vi "tsdiag_can_read_data_by_identifier.vi"(8 "error in (no error)":errorcluster, 9 "ADataIdentifier":u16 format="%.0x", 10 "ADiagModuleIndex":i32, 11 "路径输入":path) -> (0 "error out":errorcluster, 1 "Data":u8[](array[numeric]), 2 "return":i32, 3 "路径输出":path)   [LabVIEW 2014]
doc: "22服务，根据ID读取数据。"
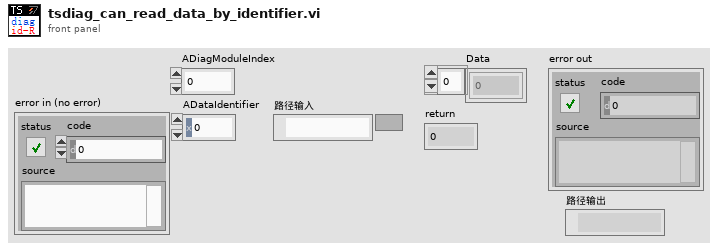
[diagram p1: front panel]
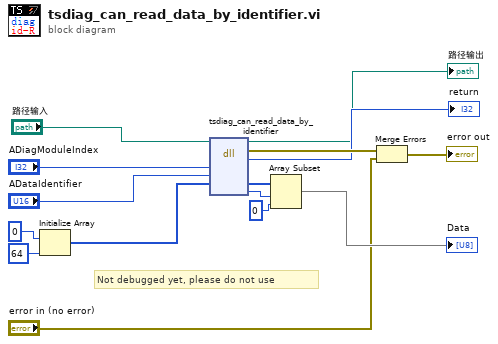
[diagram p0: block diagram]
diagram:
  # "Not debugged yet, please do not use"
  n1 = Initialize Array(u8 0, 64 ("dimension size")) -> (w9:u8[])
  n2 = dll-call lib="D:/Program Files (x86)/TOSUN/TSMaster/bin/TSMaster.dll" fn="tsdiag_can_read_data_by_identifier"(path in="路径输入", "ADiagModuleIndex"="ADiagModuleIndex", "ADataIdentifier"="ADataIdentifier", "AReturnArray"=w9) -> (path out=→"路径输出":path, error out=w15:errorcluster, "ACode"=→"return":i32, "AReturnArray"=w7:u8[], "AReturnArraySize"=w8:i32)  [unwired: 5 in]
  n3 = Array Subset(array=w7, index=w8, length=0) -> (→"Data":u8[])
  n4 = Merge Errors(w15, "error in (no error)") -> (→"error out":errorcluster)
